vi "Register for Events (Single PyObject).vi"(8 "error in (no error)":errorcluster, 9 "Functions":T1[](array[typedef]), 10 "PyObject Name":string, 11 "JKI_Python_Server in":refnum<class "Server.lvclass">) -> (0 "error out":errorcluster, 1 "Python":T2, 3 "JKI_Python_Server out":refnum<class "Server.lvclass">)   [LabVIEW 2020, in "jki_python_bridge.lvlib" / "Server.lvclass"]
uses:
  Server.lvclass
  Type Definitions/Python Method Call - Event Registration.ctl
  Call/Call.lvclass
  Type Definitions/Public Events - Cluster.ctl
  Type Definitions/Python Method.ctl
  PyObject/PyObject.lvclass
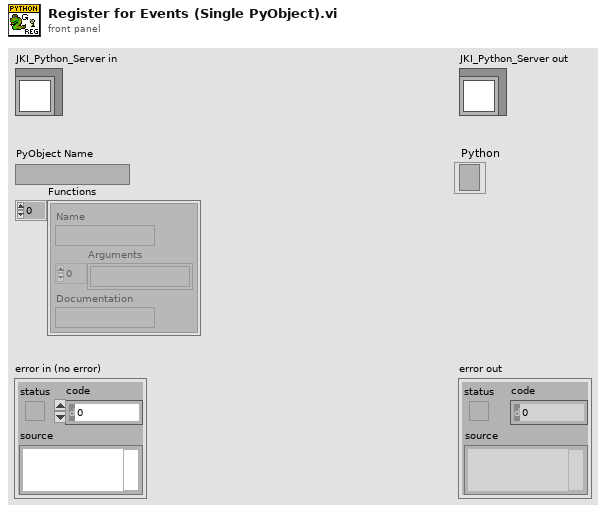
[diagram p1: front panel]
types:
  T1 = typedef "jki_python_bridge.lvlib/Server.lvclass/Python Method.ctl" = cluster{"Name":string, "Arguments":string[], "Documentation":string}
  T2 = typedef "jki_python_bridge.lvlib/Server.lvclass/Python Method Call - Event Registration.ctl" = refnum<event-registration>
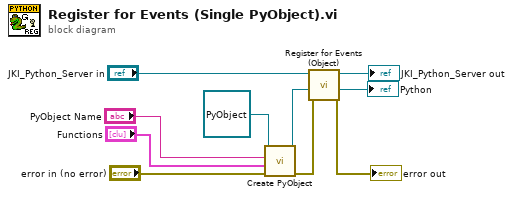
[diagram p0: block diagram]
diagram:
  n1 = call "Create PyObject.vi"("error in (no error)"="error in (no error)", "Methods"="Functions", "PyObject Name"="PyObject Name", "Node in"=refnum<class "PyObject.lvclass"> refnum) -> ("error out"=w2:errorcluster, "Node out"=w9:refnum<class "PyObject.lvclass">)  [unwired: 6 in]
  n2 = call "Register for Events (Object).vi"("error in (no error)"=w2, "PyObject.lvclass"=w9, "JKI_Python_Server in"="JKI_Python_Server in") -> ("error out"=→"error out":errorcluster, "Python Event"=→"Python":T2, "JKI_Python_Server out"=→"JKI_Python_Server out":refnum<class "Server.lvclass">)  [unwired: 6 in]
